vi "Open Recordset.vi"(4 "error in (no error)":errorcluster, 5 "Recordset Parameters":cluster{"CursorType":T1, "LockType":T2}={"CursorType"=1, "LockType"=3} {"LockType" items=["adLockUnspecified"=-1, "adLockReadOnly"=1, "adLockPessimistic"=2, "adLockOptimistic"=3, "adLockBatchOptimistic"=4]; "CursorType" items=["adOpenUnspecified"=-1, "adOpenForwardOnly"=0, "adOpenKeyset"=1, "adOpenDynamic"=2, "adOpenStatic"=3]}, 6 "Source":string, 7 "Connection":refnum<k7>) -> (0 "error out":errorcluster, 3 "Recordset":refnum<k7>)   [LabVIEW 2020, in "ADO Database Drivers.lvlib"]
uses:
  ADO Database Drivers.lvlib
  _typedefs/CursorType.ctl
  _typedefs/LockType.ctl
panel:
  in  "?":refnum<k7>
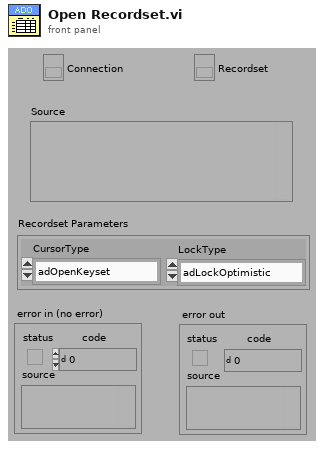
[diagram p1: front panel]
types:
  T1 = typedef "ADO Database Drivers.lvlib/CursorType.ctl" = i32
  T2 = typedef "ADO Database Drivers.lvlib/LockType.ctl" = i32
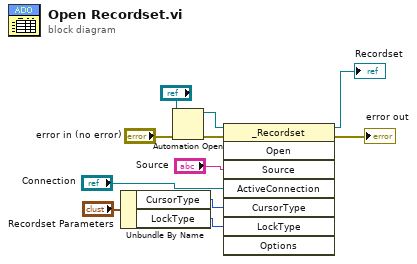
[diagram p0: block diagram]
diagram:
  n1 = Unbundle By Name("Recordset Parameters") -> ("CursorType"=w4:T1, "LockType"=w3:T2)
  n2 = Automation Open(error in (no error)="error in (no error)", Automation Refnum="?") -> (Automation Refnum=w11:refnum<k7>, error out=w9:errorcluster)  [unwired: 2 in]
  n3 = invoke class="_Recordset" method="Open"(reference=w11, error in=w9, "Source"="Source", "ActiveConnection"="Connection", "CursorType"=w4, "LockType"=w3) -> (reference out=→"Recordset":refnum<k7>, error out=→"error out":errorcluster)  [unwired: 2 in, 6 out]
